vi "choose_technique.vi"() -> (1 "technique_sequence":i32[](array[numeric]))   [LabVIEW 2014]
panel:
  in  "Technique":T1(ring)
  out "Instruction":string
  in  "OK Button":bool
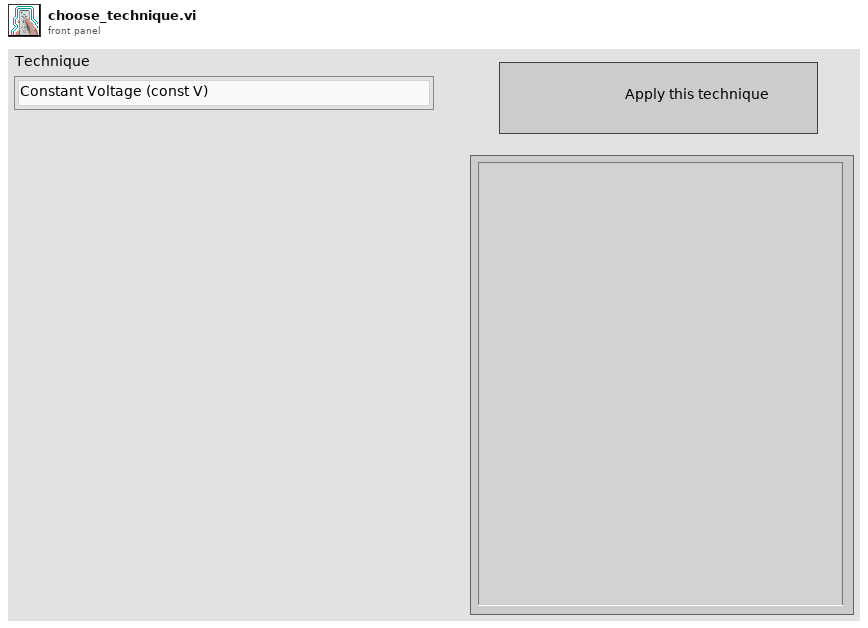
[diagram p1: front panel]
types:
  T1 = enum16{"Constant Voltage (const V)", "Cyclic Voltammetry (CV)", "Differential Pulse Voltammetry (DPV)"}
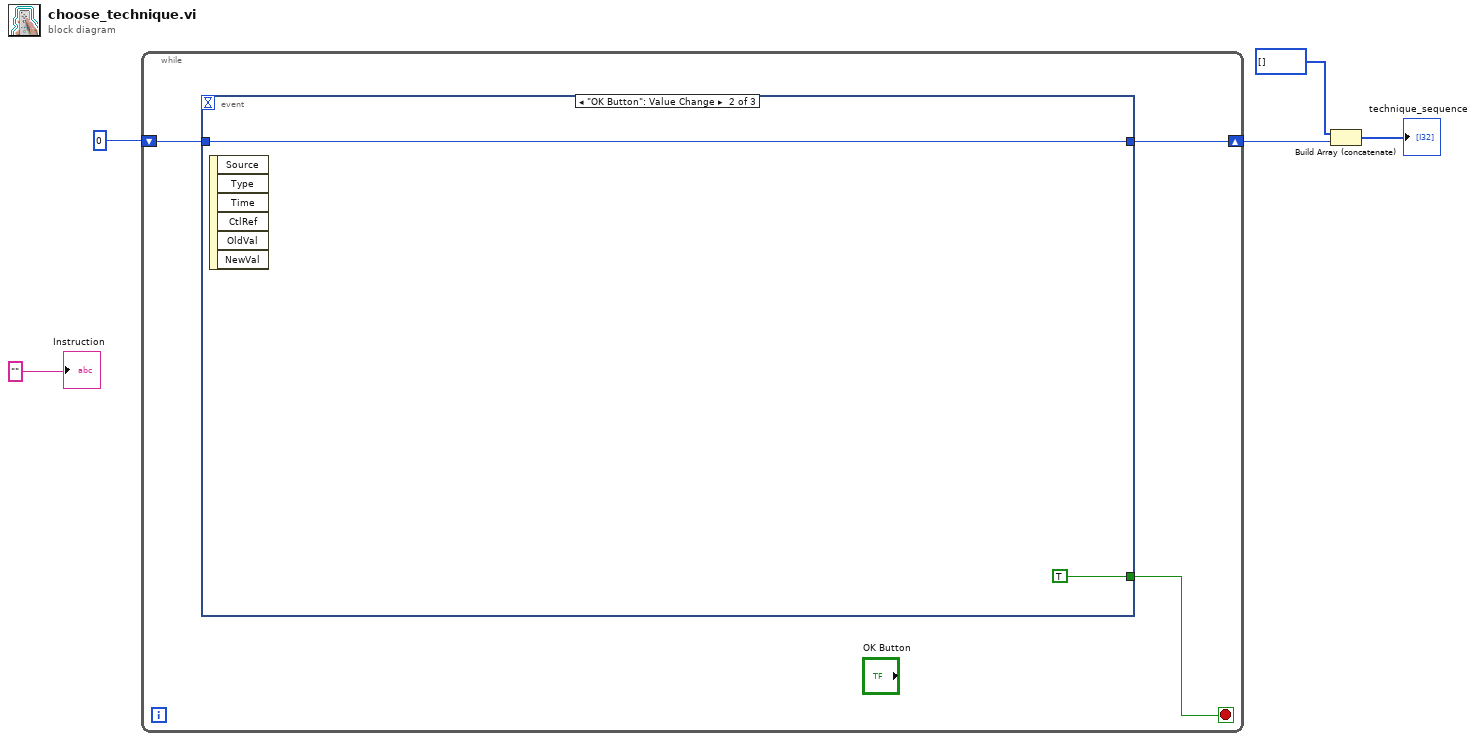
[diagram p0: block diagram]
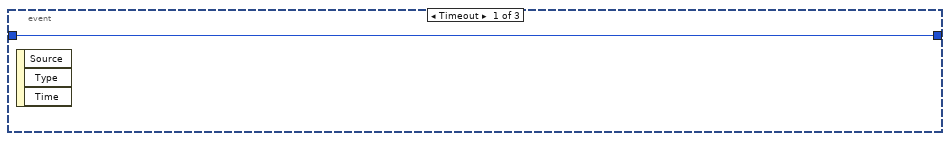
[diagram p2: hidden frame]
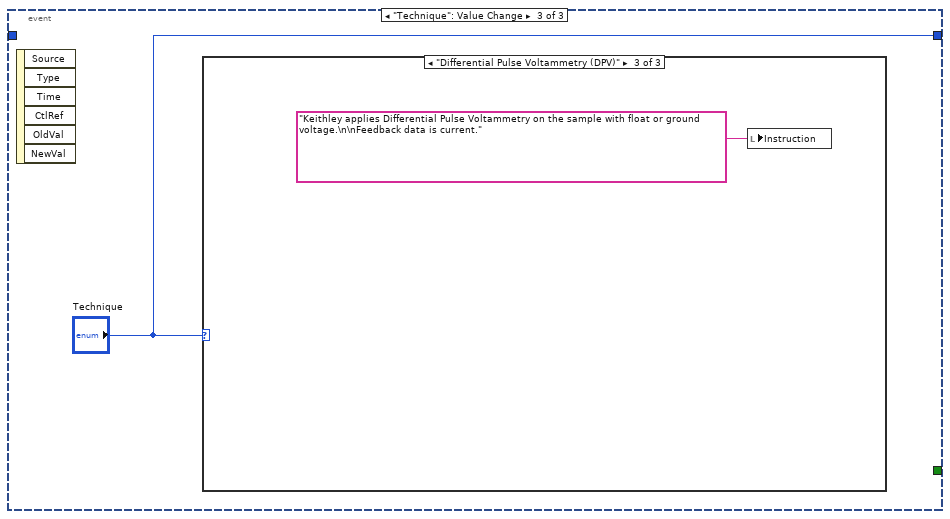
[diagram p3: hidden frame]
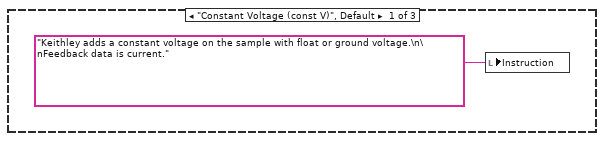
[diagram p4: hidden frame]
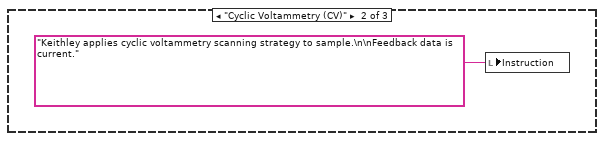
[diagram p5: hidden frame]
diagram:
  n1 = while {
    shift-right: [w7] -> w2
    shift-left: 0 -> [w6]
    stop <- w8 stop-if-true
    n2 = event shown="[1] \"OK Button\": Value Change" {
      selector: _ -> [_ _ _]
      dyn-events: _ -> [_ _ _]
      timeout: _ -> [_ _ _]
      tunnel: [_ TRUE _] -> w8
      tunnel: [w9 w10 "Technique"] -> w7
      tunnel: w6 -> [w9 w10 _]
      event Timeout {
        n3 = event-data() -> ()  [unwired: 1 in, 3 out]
      }
      event "OK Button": Value Change {
        n4 = event-data() -> ()  [unwired: 1 in, 6 out]
      }
      event "Technique": Value Change {
        n5 = event-data() -> ()  [unwired: 1 in, 6 out]
        n6 = case shown="\"Differential Pulse Voltammetry (DPV)\"" "Technique" {
          frame "Constant Voltage (const V)", Default {
            n7 = local write "Instruction"("Keithley adds a constant voltage on the sample with float or ground voltage.\n\nFeedback data is current.") -> ()
          }
          frame "Cyclic Voltammetry (CV)" {
            n8 = local write "Instruction"("Keithley applies cyclic voltammetry scanning strategy to sample.\n\nFeedback data is current.") -> ()
          }
          frame "Differential Pulse Voltammetry (DPV)" {
            n9 = local write "Instruction"("Keithley applies Differential Pulse Voltammetry on the sample with float or ground voltage.\n\nFeedback data is current.") -> ()
          }
        }
      }
    }
  }
  n10 = Build Array (concatenate)(i32[] [], w2) -> (→"technique_sequence":i32[])
  "Instruction" <- ""
